vi "Trans_Cap.vi"(11 "Read Buffer":string) -> (2 "String":string, 3 "Numeric":dbl)   [LabVIEW 2017]
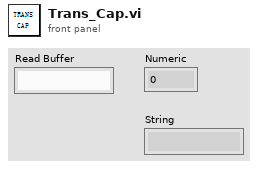
[diagram p1: front panel]
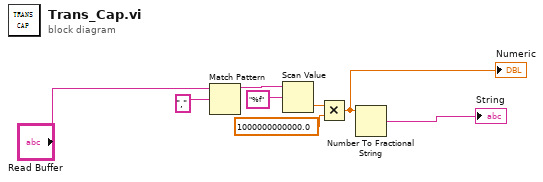
[diagram p0: block diagram]
diagram:
  n1 = Match Pattern(string="Read Buffer", regular expression=",") -> (before substring=w4:string)  [unwired: 1 in, 3 out]
  n2 = Scan Value(string=w4, format string="%f" ("格式字符串")) -> (value=w5:dbl)  [unwired: 1 in, 1 out]
  n3 = Multiply(x=w5, y=1000000000000.0) -> (x*y=w7:dbl)
  "Numeric" <- w7
  n4 = Number To Fractional String(number=w7) -> (F-format string=→"String":string)  [unwired: 3 in]
